vi "Mac2LinuxPath.vi"(8 "Error In":errorcluster, 11 "Mac Path":path) -> (0 "Error Out":errorcluster, 3 "Linux Path":string)   [LabVIEW 2010]
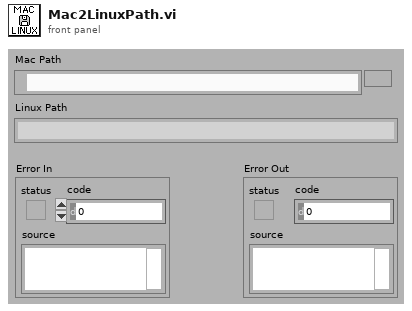
[diagram p1: front panel]
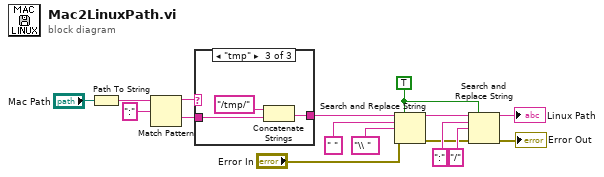
[diagram p0: block diagram]
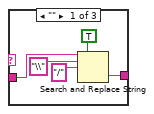
[diagram p2: hidden frame]
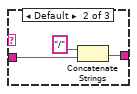
[diagram p3: hidden frame]
diagram:
  w7 = TRUE ("replace all? (F)")
  n1 = Path To String(path="Mac Path") -> (string=w5:string)
  n2 = Match Pattern(string=w5, regular expression=":") -> (before substring=w1:string, after substring=w3:string)  [unwired: 1 in, 2 out]
  n3 = case shown="\"tmp\"" w1 {
    tunnel: w3 -> [w20 w24 w27]
    tunnel: [w21 w22 w25] -> w2
    frame "" {
      n4 = Search and Replace String(replace all?=TRUE ("replace all? (F)"), input string=w20, search string="\\", replace string="/" ("replace string (\"\")")) -> (result string=w21:string)  [unwired: 4 in, 3 out]
    }
    frame Default {
      n5 = Concatenate Strings("/" ("string"), w24) -> (w22:string)
    }
    frame "tmp" {
      n6 = Concatenate Strings("/tmp/" ("string"), w27) -> (w25:string)
    }
  }
  n7 = Search and Replace String(replace all?=w7, input string=w2, search string=" ", replace string="\\ " ("replace string (\"\")"), error in="Error In") -> (result string=w14:string, error out=w10:errorcluster)  [unwired: 3 in, 2 out]
  n8 = Search and Replace String(replace all?=w7, input string=w14, search string=":", replace string="/" ("replace string (\"\")"), error in=w10) -> (result string=→"Linux Path":string, error out=→"Error Out":errorcluster)  [unwired: 3 in, 2 out]
